vi "Weighted Array Median.vi"(8 "Error In":errorcluster, 9 "Weight Array":dbl[](array[numeric]), 11 "X Array":dbl[](array[numeric])) -> (0 "Error Out":errorcluster, 1 "Weighted":bool, 3 "Median":dbl)   [LabVIEW 2021, in "Math.lvlib"]
uses:
  fa00327a-ba96-4286-85e6-9327a8432af6.vi
  a0bdc1c7-d0ee-4143-aa97-a44ed1202da8.vi
  fd33fecc-40ae-4180-84de-07ed15a0d76e.vi
  fa00327a-ba96-4286-85e6-9327a8432af6.vi/b4ed6f1f-2671-4a60-8569-53a663278391.vi
  fa00327a-ba96-4286-85e6-9327a8432af6.vi/b4ed6f1f-2671-4a60-8569-53a663278391.vi/59314c09-68ff-4b78-8684-0242d4040ca4.vi
  fa00327a-ba96-4286-85e6-9327a8432af6.vi/b4ed6f1f-2671-4a60-8569-53a663278391.vi/59314c09-68ff-4b78-8684-0242d4040ca4.vi/d4db2432-cc9c-482c-8957-dac855435ef6.vi
  fa00327a-ba96-4286-85e6-9327a8432af6.vi/b4ed6f1f-2671-4a60-8569-53a663278391.vi/59314c09-68ff-4b78-8684-0242d4040ca4.vi/86fbf154-bd7b-49a2-8ab2-a837b2a95f24.vi
  fa00327a-ba96-4286-85e6-9327a8432af6.vi/b4ed6f1f-2671-4a60-8569-53a663278391.vi/59314c09-68ff-4b78-8684-0242d4040ca4.vi/3b95b01e-1ec2-4565-bcd9-7606a5281010.vi
  fa00327a-ba96-4286-85e6-9327a8432af6.vi/b4ed6f1f-2671-4a60-8569-53a663278391.vi/59314c09-68ff-4b78-8684-0242d4040ca4.vi/96a08935-737a-44b2-979c-a81d56408f7e.vi
  fa00327a-ba96-4286-85e6-9327a8432af6.vi/b4ed6f1f-2671-4a60-8569-53a663278391.vi/59314c09-68ff-4b78-8684-0242d4040ca4.vi/d4db2432-cc9c-482c-8957-dac855435ef6.vi/6eaecd13-6e48-4772-a921-b51ebdf84d88.vi
  fa00327a-ba96-4286-85e6-9327a8432af6.vi/b4ed6f1f-2671-4a60-8569-53a663278391.vi/59314c09-68ff-4b78-8684-0242d4040ca4.vi/d4db2432-cc9c-482c-8957-dac855435ef6.vi/d2d5f2b7-06f4-47f6-971c-049c3fdbb653.vi
  fa00327a-ba96-4286-85e6-9327a8432af6.vi/b4ed6f1f-2671-4a60-8569-53a663278391.vi/59314c09-68ff-4b78-8684-0242d4040ca4.vi/3b95b01e-1ec2-4565-bcd9-7606a5281010.vi/6eaecd13-6e48-4772-a921-b51ebdf84d88.vi
  fa00327a-ba96-4286-85e6-9327a8432af6.vi/b4ed6f1f-2671-4a60-8569-53a663278391.vi/59314c09-68ff-4b78-8684-0242d4040ca4.vi/3b95b01e-1ec2-4565-bcd9-7606a5281010.vi/d2d5f2b7-06f4-47f6-971c-049c3fdbb653.vi
  fa00327a-ba96-4286-85e6-9327a8432af6.vi/b4ed6f1f-2671-4a60-8569-53a663278391.vi/59314c09-68ff-4b78-8684-0242d4040ca4.vi/96a08935-737a-44b2-979c-a81d56408f7e.vi/6eaecd13-6e48-4772-a921-b51ebdf84d88.vi
  fa00327a-ba96-4286-85e6-9327a8432af6.vi/b4ed6f1f-2671-4a60-8569-53a663278391.vi/59314c09-68ff-4b78-8684-0242d4040ca4.vi/96a08935-737a-44b2-979c-a81d56408f7e.vi/d2d5f2b7-06f4-47f6-971c-049c3fdbb653.vi
  <userlib>/_OpenG.lib/array/array.llb/Sort 1D Array (DBL)__ogtk.vi
  <userlib>/_OpenG.lib/array/array.llb/Reorder 1D Array2 (DBL)__ogtk.vi
  Arrays/Signed Array Index.vi
  <vilib>/Comparison/Less/Less Functor/Less Functor.lvclass
  Math.lvlib
  <userlib>/_OpenG.lib/array/array.llb/openg_array.lvlib
panel:
  # "see the License on the block diagram (Ctrl+E or Window:Show Block Diagram)"
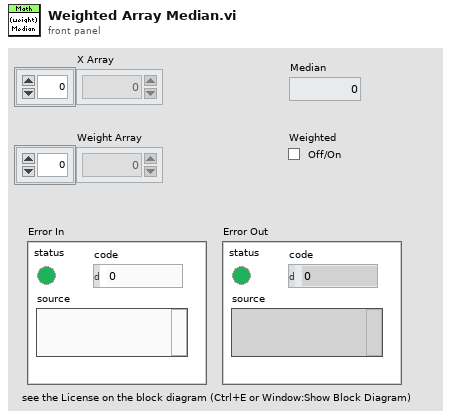
[diagram p1: front panel]
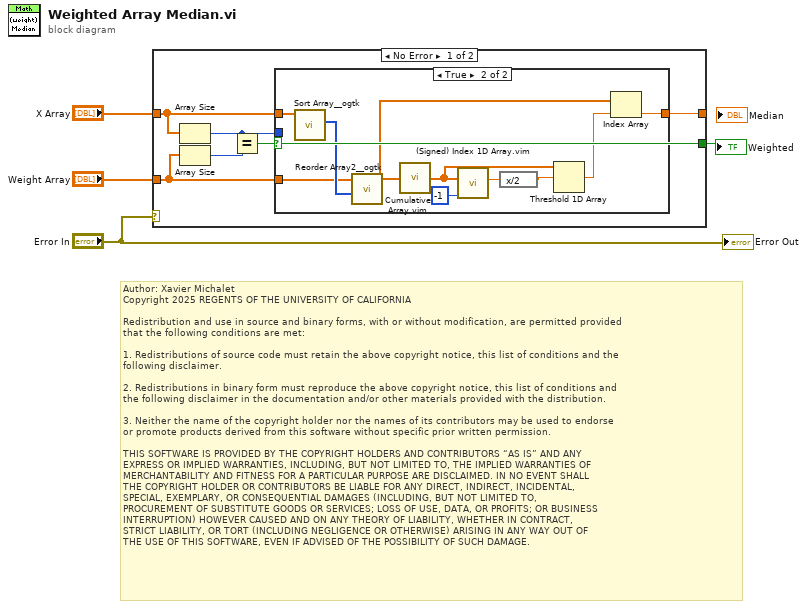
[diagram p0: block diagram]
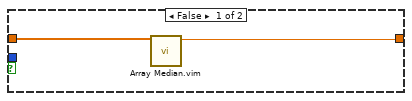
[diagram p2: hidden frame]
diagram:
  # "Author: Xavier Michalet\nCopyright 2025 REGENTS OF THE UNIVERSITY OF CALIFORNIA\n\nRedistribution and use in source and binary forms, with or without modification, are permitted provided\nthat the following conditions are met:\n\n1. Redistributions of source code must retain the above copyright notice, this list of conditions and the\nfollowing disclaimer.\n\n2. Redistributions in binary form must reproduce the above copyright notice, this list of conditions and\nthe following disclaimer in the documentation and/or other materials provided with the distribution.\n\n3. Neither the name of the copyright holder nor the names of its contributors may be used to endorse \nor promote products derived from this software without specific prior written permission.\n\nTHIS SOFTWARE IS PROVIDED BY THE COPYRIGHT HOLDERS AND CONTRIBUTORS “AS IS” AND ANY \nEXPRESS OR IMPLIED WARRANTIES, INCLUDING, BUT NOT LIMITED TO, THE IMPLIED WARRANTIES OF\nMERCHANTABILITY AND FITNESS FOR A PARTICULAR PURPOSE ARE DISCLAIMED. IN NO EVENT SHALL\nTHE COPYRIGHT HOLDER OR CONTRIBUTORS BE LIABLE FOR ANY DIRECT, INDIRECT, INCIDENTAL, \nSPECIAL, EXEMPLARY, OR CONSEQUENTIAL DAMAGES (INCLUDING, BUT NOT LIMITED TO, \nPROCUREMENT OF SUBSTITUTE GOODS OR SERVICES; LOSS OF USE, DATA, OR PROFITS; OR BUSINESS\nINTERRUPTION) HOWEVER CAUSED AND ON ANY THEORY OF LIABILITY, WHETHER IN CONTRACT, \nSTRICT LIABILITY, OR TORT (INCLUDING NEGLIGENCE OR OTHERWISE) ARISING IN ANY WAY OUT OF\nTHE USE OF THIS SOFTWARE, EVEN IF ADVISED OF THE POSSIBILITY OF SUCH DAMAGE."
  n1 = case shown="No Error" "Error In" {
    tunnel: "X Array" -> [w9 _]
    tunnel: "Weight Array" -> [w8 _]
    tunnel: [w5 _] -> _
    tunnel: [w6 _] -> w1
    frame No Error {
      n2 = Array Size(array=w9) -> (size(s)=w7:i32)
      n3 = Array Size(array=w8) -> (size(s)=w10:i32)
      n4 = Equal?(x=w7, y=w10) -> (x = y?=w6:bool)
      n5 = case shown="True" w6 {
        tunnel: w9 -> [w12 w22]
        tunnel: w8 -> [_ w16]
        tunnel: [w11 w13] -> w5
        tunnel: w7 -> [_ _]
        frame False {
          n6 = call "Array Median.vim"("Array"=w12) -> ("Median"=w11:dbl)  [unwired: 10 in]
        }
        frame True {
          n7 = call-poly <userlib>:"Sort Array__ogtk.vi"("Array in"=w22) -> ("Sorted Pointers"=w21:i32[])  [unwired: 9 in, 1 out]
          n8 = call-poly <userlib>:"Reorder Array2__ogtk.vi"("indices"=w21, "array"=w16) -> ("reordered array"=w15:dbl[])  [unwired: 9 in]
          n9 = call "Cumulative Array.vim"("Array"=w15) -> ("cumulative Array"=w17:dbl[])  [unwired: 8 in]
          n10 = call "(Signed) Index 1D Array.vim"("Signed Index"=-1, "Array"=w17) -> ("Array Element"=w19:dbl)  [unwired: 9 in]
          n11 = expression code="x/2"(w19) -> (w18:dbl)
          n12 = Threshold 1D Array(2:w18, 3:w17) -> (0:w14:dbl)  [unwired: 1 in]
          n13 = Index Array(array=w15, index=w14) -> (element=w13:dbl)
        }
      }
    }
    frame Error {
    }
  }
  "Weighted" <- w1
  "Error Out" <- "Error In"
